vi "ask_model.vi"(0 "agent_simple_qa in":refnum<class "agent_simple_qa.lvclass">, 5 "message_text":refnum<class "message_text.lvclass">, 11 "error in (no error)":errorcluster) -> (4 "agent_simple_qa out":refnum<class "agent_simple_qa.lvclass">, 6 "message_text_response":refnum<class "message_text.lvclass">, 15 "error out":errorcluster)   [LabVIEW 2020, in "agent_simple_qa.lvclass"]
uses:
  agent_simple_qa.lvclass
  models/message_text/message_text.lvclass
  D:/petwork/labview-llm-libraries/src/models/abstract_message_base/abstract_message_base.lvclass
  agent_simple_qa.lvclass/agent_simple_qa.ctl
  models/abstract_llm_chatcompletion/abstract_llm_chatcompletion.lvclass
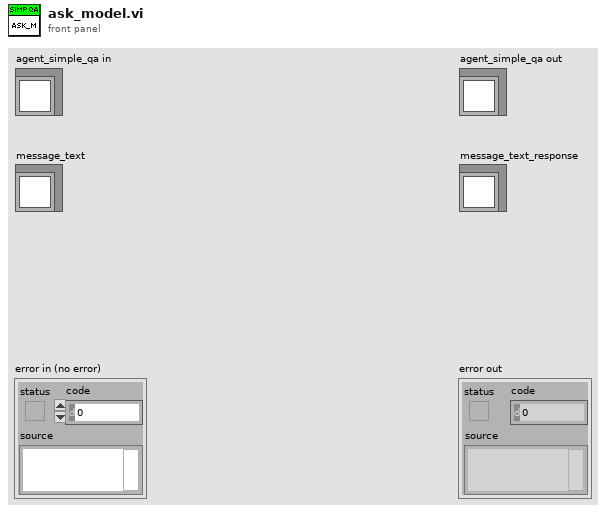
[diagram p1: front panel]
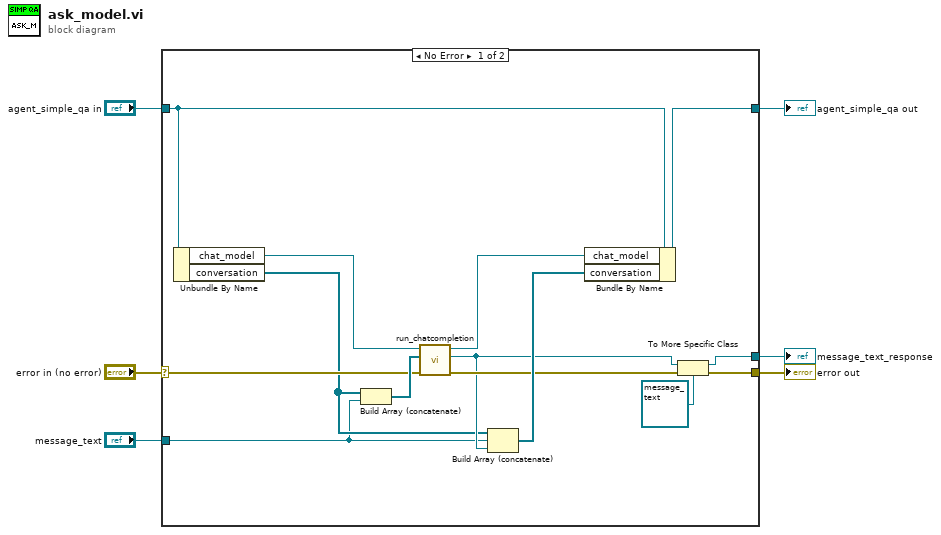
[diagram p0: block diagram]
diagram:
  n1 = case shown="No Error" "error in (no error)" {
    selector: "error in (no error)" -> [w11 w22]
    tunnel: [w15 w22] -> w5
    tunnel: [w19 w21] -> w3
    tunnel: "agent_simple_qa in" -> [w9 w21]
    tunnel: "message_text" -> [w7 _]
    tunnel: [w12 _] -> w1
    frame No Error {
      n2 = Unbundle By Name(w9) -> ("chat_model"=w10:refnum<class "abstract_llm_base.lvclass">, "conversation"=w8:refnum<class "abstract_message_base.lvclass">[])
      n3 = Build Array (concatenate)(w8, w7) -> (w18:refnum<class "abstract_message_base.lvclass">[])
      n4 = call "run_chatcompletion.vi"("error in (no error)"=w11, "Messages"=w18, "abstract_llm_chatcompletion in"=w10) -> ("error out"=w16:errorcluster, "Response"=w14:refnum<class "abstract_message_base.lvclass">, "abstract_llm_chatcompletion out"=w20:refnum<class "abstract_llm_base.lvclass">)  [unwired: 6 in]
      n5 = Build Array (concatenate)(w8, w7, w14) -> (w17:refnum<class "abstract_message_base.lvclass">[])
      n6 = Bundle By Name(cluster=w9, "chat_model"=w20, "conversation"=w17) -> (w19:refnum<class "agent_simple_qa.lvclass">)
      n7 = To More Specific Class(target class=refnum<class "message_text.lvclass"> refnum ("message_text"), reference=w14, error in=w16) -> (specific class reference=w12:refnum<class "message_text.lvclass">, error out=w15:errorcluster)
    }
    frame Error {
    }
  }
  "error out" <- w5
  "agent_simple_qa out" <- w3
  "message_text_response" <- w1
